vi "sim_signal.vi"(1 "n Signals":i32=26) -> (0 "Waveform Graph":dynamicdata(graph))   [LabVIEW 2017]
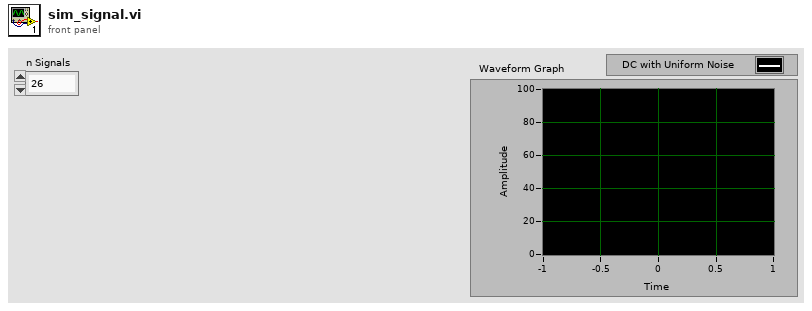
[diagram p1: front panel]
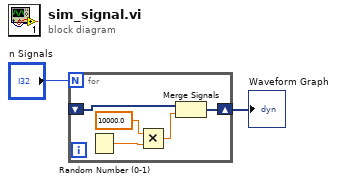
[diagram p0: block diagram]
diagram:
  n1 = for {
    N: "n Signals" -> [_]
    shift-right: [w7] -> w1
    shift-left: _ -> [w6]
    n2 = Random Number (0-1)() -> (number: 0 to 1=w4:dbl)
    n3 = Multiply(x=10000.0, y=w4) -> (x*y=w3:dbl)
    n4 = Merge Signals(w6, w3) -> (w7:dynamicdata)
  }
  "Waveform Graph" <- w1
